vi "Programa Vent.vi"() -> ()   [LabVIEW 2021]
uses:
  TabControl.ctl
  4c7040a6-f012-4fa6-bc11-eaa48d4a9fce.vi
  <vilib>/Utility/file.llb/Write Delimited Spreadsheet (DBL).vi
  <vilib>/Instr/_visa.llb/VISA Configure Serial Port (Instr).vi
panel:
  out "Fecha y Hora":timestamp=timestamp(3714054510.5922894 s since 1904-01-01) format="%<%X\n%x>T"
  in  "Modo Operación":bool=TRUE
  in  "Comenzar Respiración":bool
  in  "Modo Asistido":bool
  in  "stop":bool
  in  "Tab Control 2":T1
  out "MV":i16=211
  out "PEEP":i16=4
  out "FLUJO":i16
  out "VOLUMEN":i16=211
  in  "Porcentaje \nde flujo (%)":i32=55 min=0 max=100 step=1
  in  "PEEP":i32 min=0 max=20 step=1
  in  "Presión de Soporte":i32=15 min=10 max=60 step=1
  in  "Volumen":i32=350 min=100 max=2000 step=10
  in  "Tiempo Plateau":i32=500 min=0 max=1 step=1
  in  "Tiempo Espiración":i32=3 min=1 max=10 step=1
  out "PRESIÓN":waveform(dbl)(graph)
  out "T. CICLO":dbl=9.2 format="%#_2g"
  out "BPM":i16=7
  out "PIP":i16=1
  out "FLUJO":waveform(dbl)(graph)
  in  "(PC) Tiempo de inspiración":i32=3 min=1 max=10 step=1
  out "FLUJO 2":waveform(dbl)(graph)
  out "PRESIÓN 2":waveform(dbl)(graph)
  out "DiffPres":waveform(dbl)(graph)
  in  "PWM":bool
  in  "PEEP":bool
  in  "PRESIÓN":bool
  in  "Data storage":bool
  out "Serial Read":string="Presion: 1.42,Peep: 3.57,Presion_soporte: 20,Flujo: -0.35,Volumen deseado: 350, Volumen inspiracion: 211.01,PIP: 1.00,VEF: 1.00,VIF: 211.00,T_muestreo: 4.00, PWM Out: 5000, Timer_Count_0: 0, Etapa_Res: 0, Derivada_Presion: 0.00, duracion_ciclo: 9200.00, BPM: 6.52, PWM_Caract: 0, T. Trans_Caract: 0.00, MV: 0.00, String: 0.000000,50.000000,20.000000,5.000000,350.000000,3000.000000,500.000000,0.000000,0.000000,0.000000,0.000000\r\r\n"
  out "Serial Write":string="0.000000,50.000000,20.000000,5.000000,350.000000,3000.000000,500.000000,0.000000,0.000000,0.000000,0.000000\r\n"
  in  "Caract. Escalon":bool
  in  "Caract. Rampa":bool
  in  "Comenzar Caracterizacion":bool
  in  "KI":i32=45 min=0 max=100 step=1
  in  "KP":i32=100 min=0 max=1000 step=1
  out "TIEMPO \nDE CICLO":dbl
  out "PRESIÓN SOPORTE\n (DEBUGGING)":dbl
  out "ETAPA \nRESPIRATORIA":dbl
  out "ERROR (PC)":dbl
  out "PWM \nCARACTERIZACIÓN":dbl
  out "PWM OUT":dbl
  in  "Caract. Pulmón":bool
  in  "Ruta de archivo":path=path "C:/Users/arakh/Desktop/MejoraVI/CalibTeensy.txt"
  in  "PRESIÓN MAX.":i32=30 min=0 max=100 step=1
  in  "PEEP MAX.":i32=30 min=0 max=100 step=1
  in  "RAPIDEZ APERTURA %":i32=30 min=0 max=100 step=1
  out "DeltaPDecay":waveform(dbl)(graph)
  out "PWM Out":waveform(dbl)(graph)
  # "Modo de Operación"
  # "INICIO"
  # "Funciones"
  # "GRÁFICOS"
  # "AJUSTES"
  # "AVANZADO"
  # "Ventilador Mecánico de Emergencia UTP-100P v5"
  # "PARÁMETROS FUNCIONALES"
  # "Porcentaje \nde flujo (%)"
  # "PEEP\n (cm H2O)"
  # "GRÁFICOS"
  # "PC: Tiempo de insp.  (seg.)"
  # "Presión de \nsoporte \n(cm H2O)"
  # "Volumen(ml)"
  # "Tiempo de esp. (seg.)"
  # "Tiempo de plateau (miliseg.)"
  # "tiempo"
  # "GRÁFICOS"
  # "PRESIÓN (cm H20)"
  # "Tiempo"
  # "AJUSTES"
  # "CARACTERIZACIÓN\n DE VÁLVULA"
  # "(PC) AJUSTES DE CONTROLADOR"
  # "ALMACENAMIENTO\nDE DATOS"
  # "CARACTERIZACIÓN \nDE PULMÓN"
  # "* Varía los parámetros incrementalmente por cada ciclo respiratorio."
  # "DATOS TEENSY"
  # "Seccion de Datos:"
  # "AJUSTES AVANZADOS"
  # "Delta P Decay (Diff)"
  # "PWM out"
  # "Tiempo"
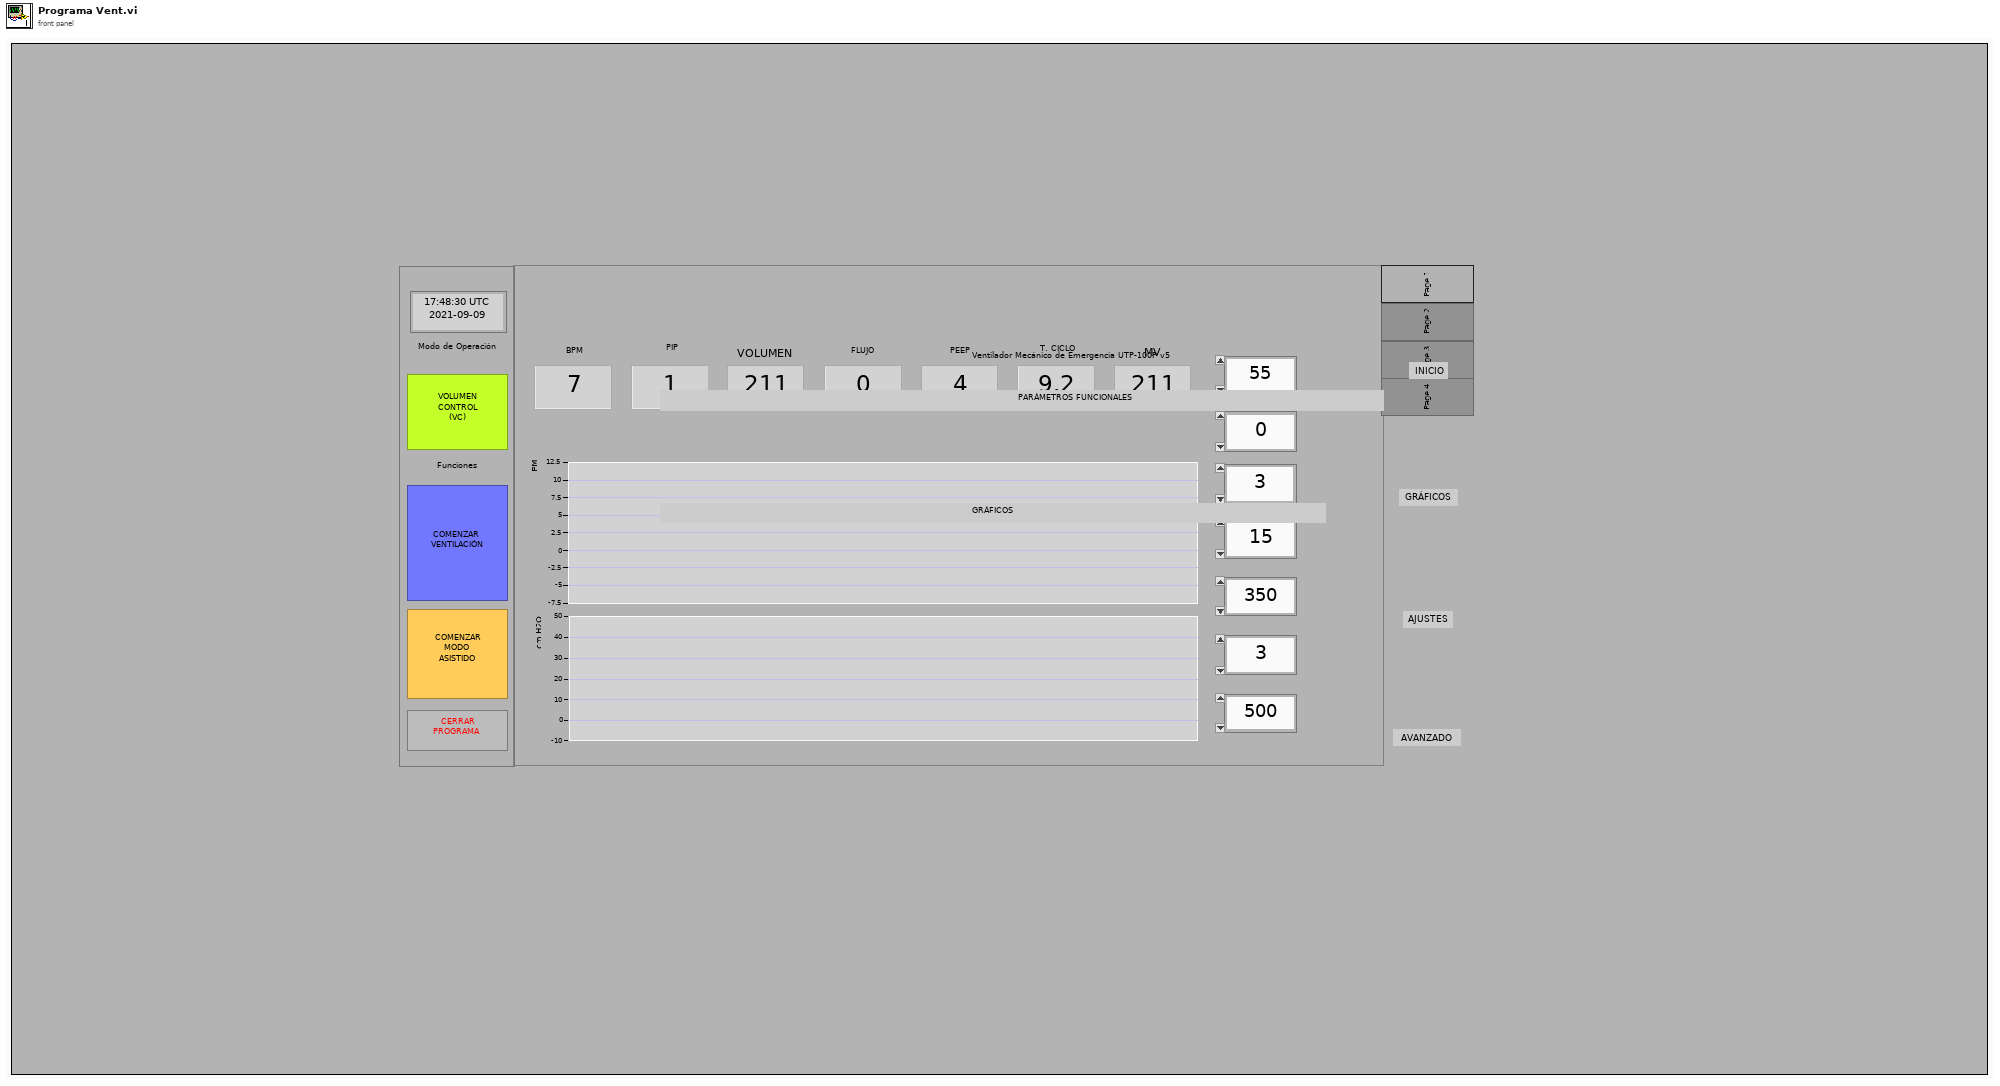
[diagram p1: front panel]
types:
  T1 = typedef "TabControl.ctl" = enum32{"Page 1", "Page 2", "Page 3", "Page 4"}
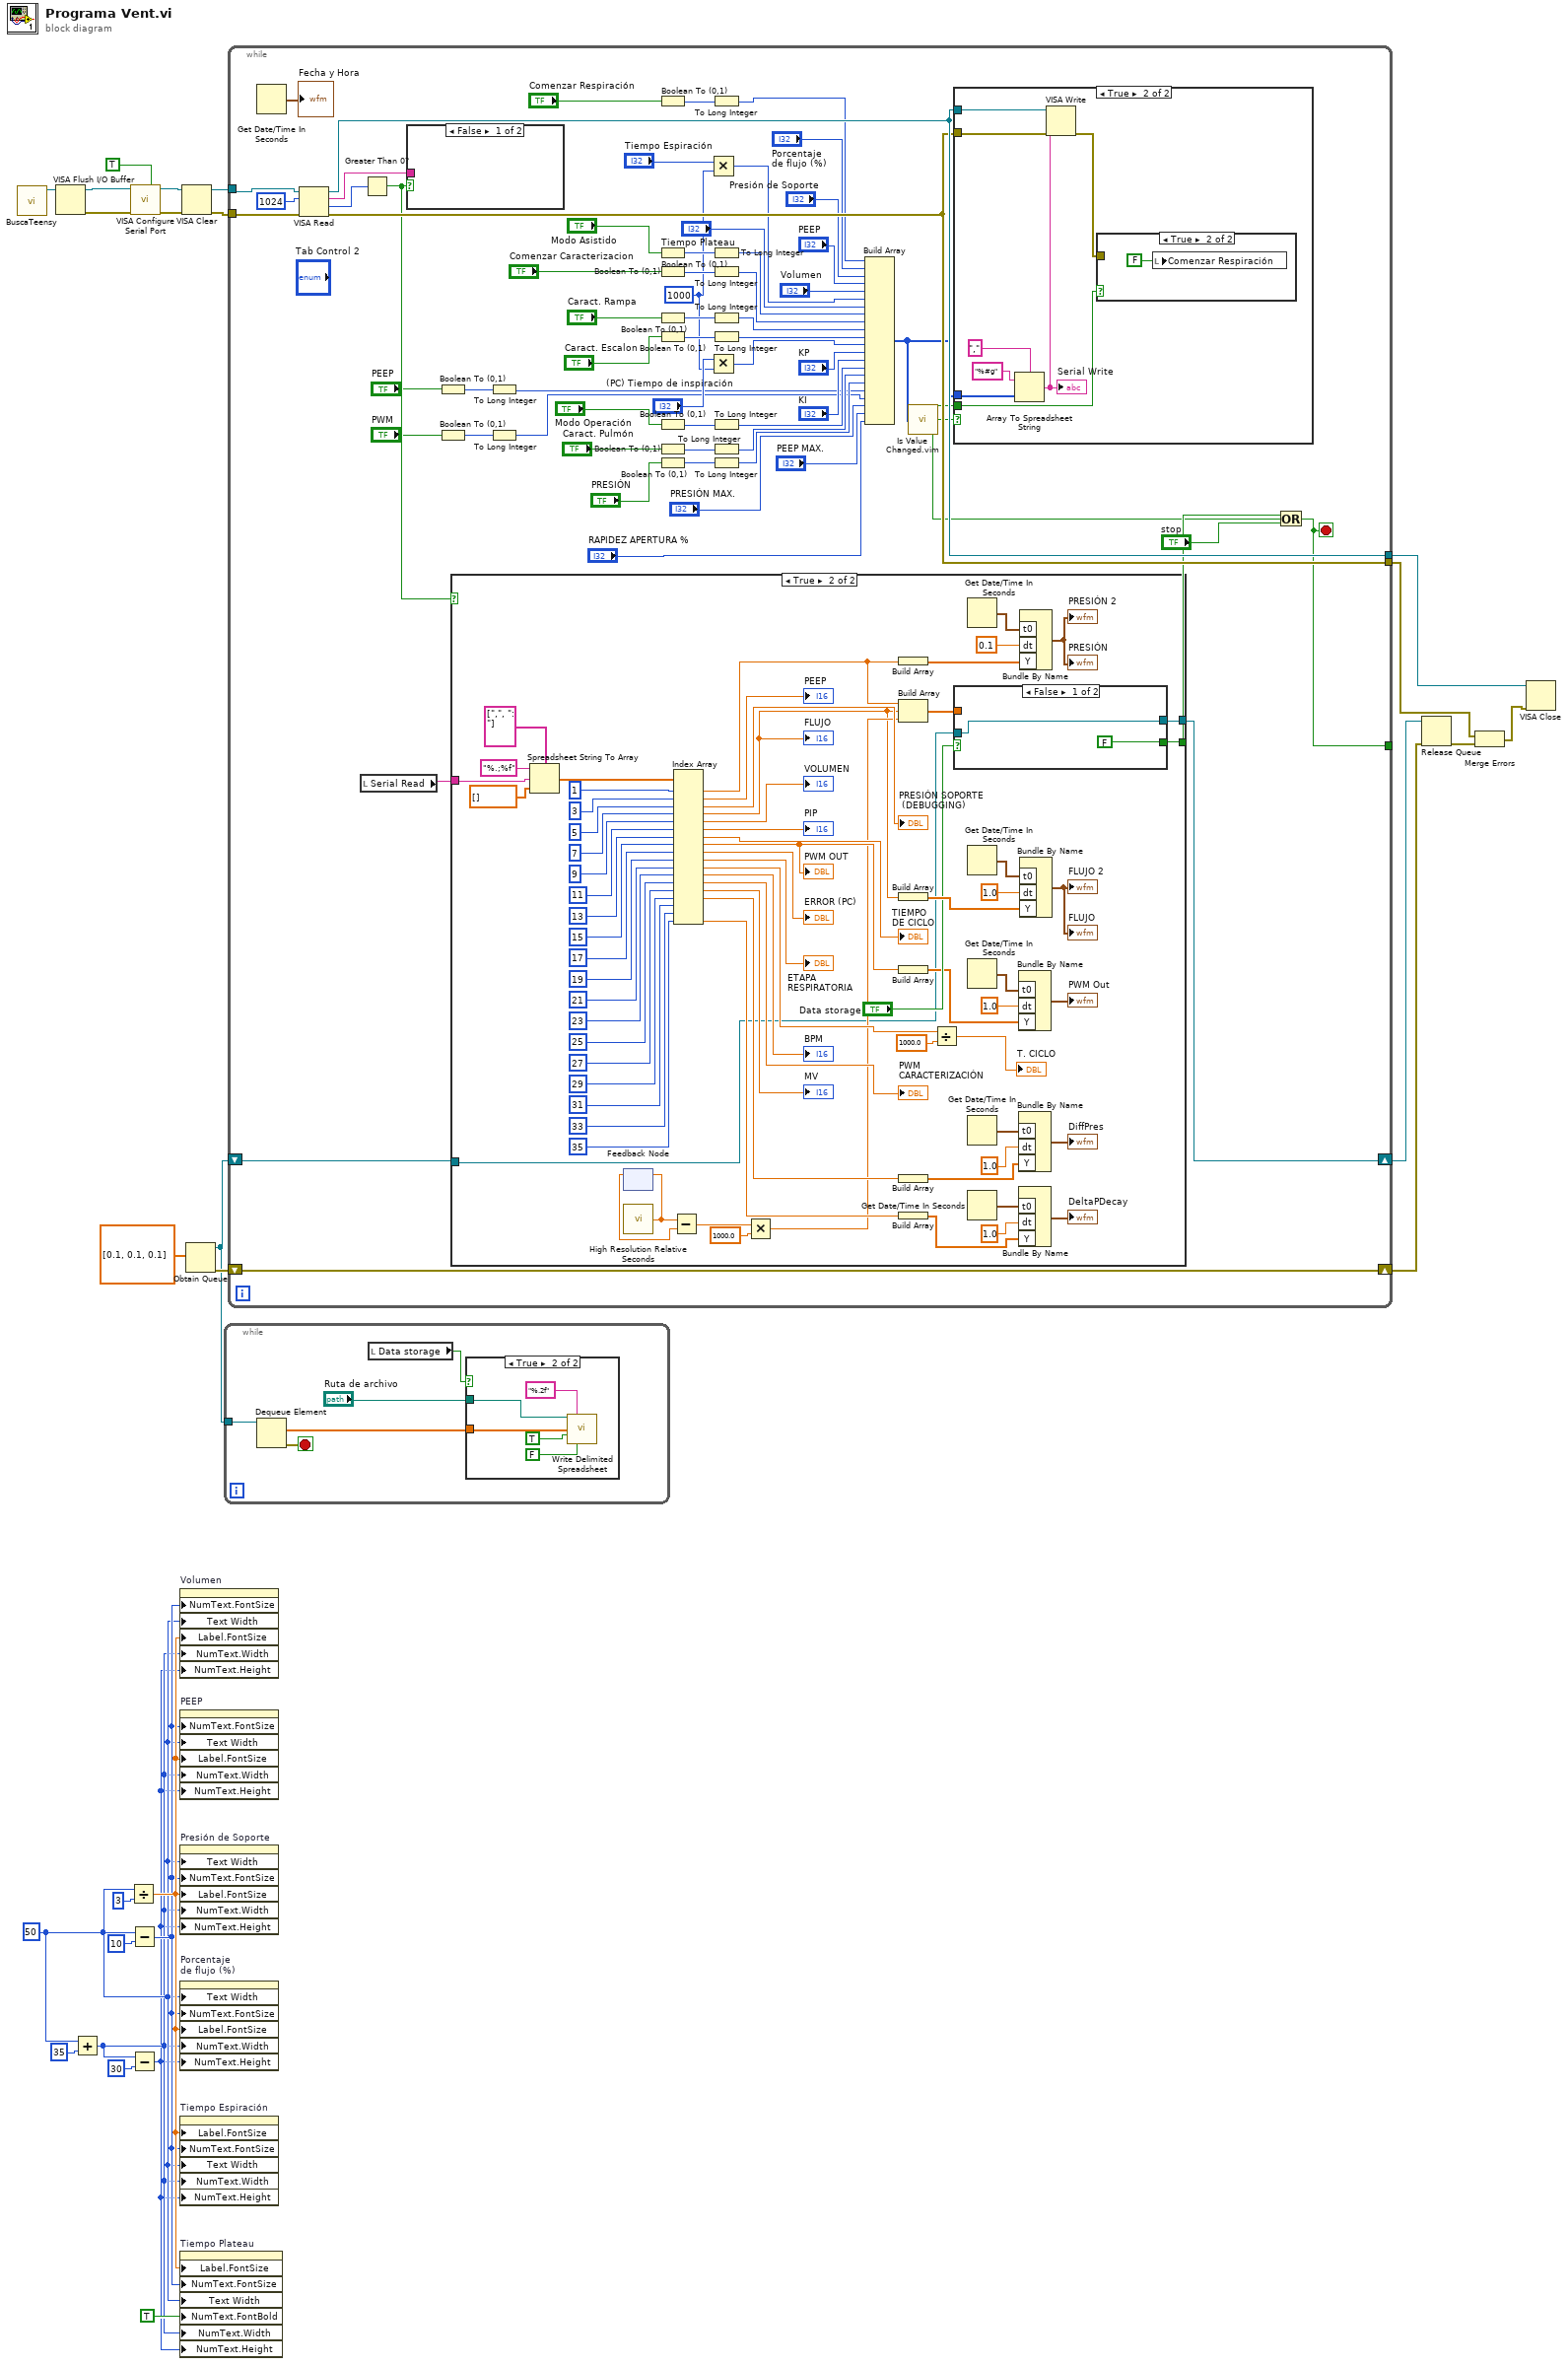
[diagram p0: block diagram]
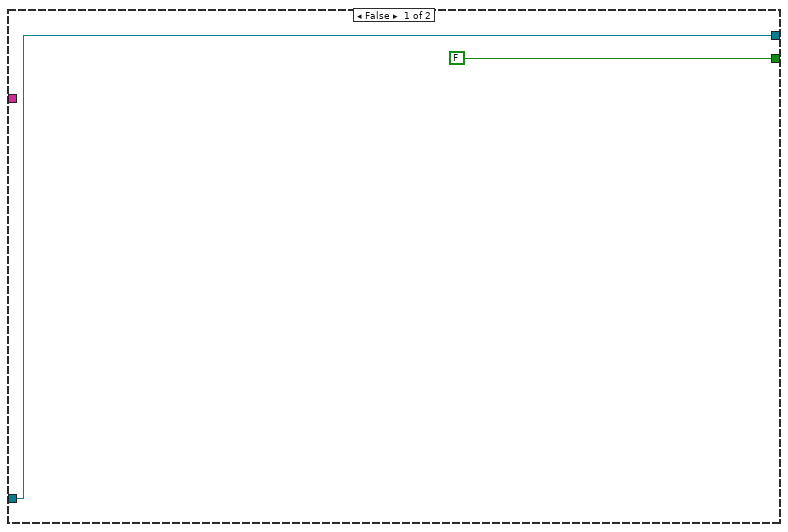
[diagram p3: hidden frame]
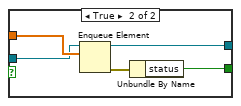
[diagram p4: hidden frame]
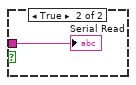
[diagram p5: hidden frame]
diagram:
  w14 = u32 50 ("Numeric Text.Size:Height")
  n1 = call "BuscaTeensy.vi"() -> ("VISA resource name out"=w19:refnum<visa-resource-name>)  [unwired: 15 in]
  n2 = VISA Flush I/O Buffer(VISA resource name=w19) -> (VISA resource name out=w21:refnum<visa-resource-name>, error out=w20:errorcluster)  [unwired: 2 in]
  n3 = Add(x=w14, y=u32 35) -> (x+y=w12:u32)
  n4 = Divide(x=w14, y=u32 3) -> (x/y=w16:dbl)
  n5 = Subtract(x=w14, y=u32 10 ("x")) -> (x-y=w15:u32)
  n6 = Subtract(x=w12, y=u32 30) -> (x-y=w10:u32)
  n7 = call-poly "VISA Configure Serial Port"("VISA resource name"=w21, "Enable Termination\nChar (T)"=TRUE ("Enable Termination\nChar (T)"), "error in (no error)"=w20) -> ("VISA resource name out"=w25:refnum<visa-resource-name>, "error out"=w24:errorcluster)  [unwired: 11 in]
  n8 = property on="Volumen" class="DigNum (strict)"("NumText.FontSize"=w15, "Text Width"=w14, "Label.FontSize"=w16, "NumText.Width"=w12, "NumText.Height"=w10) -> ()  [unwired: 2 in, 2 out]
  n9 = property on="PEEP" class="DigNum (strict)"("NumText.FontSize"=w15, "Text Width"=w14, "Label.FontSize"=w16, "NumText.Width"=w12, "NumText.Height"=w10) -> ()  [unwired: 2 in, 2 out]
  n10 = property on="Presión de Soporte" class="DigNum (strict)"("Text Width"=w14, "NumText.FontSize"=w15, "Label.FontSize"=w16, "NumText.Width"=w12, "NumText.Height"=w10) -> ()  [unwired: 2 in, 2 out]
  n11 = property on="Porcentaje \nde flujo (%)" class="DigNum (strict)"("Text Width"=w14, "NumText.FontSize"=w15, "Label.FontSize"=w16, "NumText.Width"=w12, "NumText.Height"=w10) -> ()  [unwired: 2 in, 2 out]
  n12 = property on="Tiempo Espiración" class="DigNum (strict)"("Label.FontSize"=w16, "NumText.FontSize"=w15, "Text Width"=w14, "NumText.Width"=w12, "NumText.Height"=w10) -> ()  [unwired: 2 in, 2 out]
  n13 = property on="Tiempo Plateau" class="DigNum (strict)"("Label.FontSize"=w16, "NumText.FontSize"=w15, "Text Width"=w14, "NumText.FontBold"=TRUE ("Numeric Text.Font:Bold"), "NumText.Width"=w12, "NumText.Height"=w10) -> ()  [unwired: 2 in, 2 out]
  n14 = VISA Clear(VISA resource name=w25, error in (no error)=w24) -> (VISA resource name out=w23:refnum<visa-resource-name>, error out=w22:errorcluster)
  n15 = Obtain Queue(element data type=dbl[] [0.1, 0.1, 0.1]) -> (queue out=w4:refnum<queue>, error out=w6:errorcluster)  [unwired: 4 in, 1 out]
  n16 = while {
    tunnel: w4 -> [w29]
    stop <- w30 stop-if-true
    n17 = Dequeue Element(queue=w29) -> (element=w31:dbl[], error out=w30:errorcluster)  [unwired: 2 in, 2 out]
    n18 = local read "Data storage"() -> (w32:bool)
    n19 = case shown="True" w32 {
      tunnel: w31 -> [_ w34]
      tunnel: "Ruta de archivo" -> [_ w33]
      frame False {
      }
      frame True {
        n20 = call-poly <vilib>:"Write Delimited Spreadsheet.vi"("file path (dialog if empty)"=w33, "format (%.3f)"="%.2f", "1D data"=w34, "append to file? (new file:F)"=TRUE, "transpose? (no:F)"=FALSE) -> ()  [unwired: 9 in, 2 out]
      }
    }
  }
  n21 = while {
    tunnel: [w98] -> w26
    tunnel: [w97] -> w2
    tunnel: w23 -> [w96]
    tunnel: w22 -> [w95]
    tunnel: [w40] -> _
    shift-right: [w39] -> w5
    shift-left: w6 -> [w39]
    shift-right: [w43] -> w7
    shift-left: w4 -> [w44]
    stop <- w40 stop-if-true
    w69 = 1000 ("y")
    n22 = Get Date/Time In Seconds() -> (seconds since 1Jan1904=→"Fecha y Hora":timestamp)
    n23 = VISA Read(VISA resource name=w96, byte count=u32 1024, error in (no error)=w95) -> (VISA resource name out=w98:refnum<visa-resource-name>, read buffer=w100:string, return count=w93:u32, error out=w97:errorcluster)
    n24 = local read "Serial Read"() -> (w99:string)
    n25 = Greater Than 0?(x=w93) -> (x > 0?=w92:bool)
    n26 = case shown="False" w92 {
      tunnel: w100 -> [_ w181]
      frame False {
      }
      frame True {
        "Serial Read" <- w181
      }
    }
    n27 = Boolean To (0,1)(Boolean="PEEP") -> (0, 1=w53:i16)
    n28 = Boolean To (0,1)(Boolean="PWM") -> (0, 1=w52:i16)
    n29 = case shown="True" w92 {
      tunnel: w99 -> [_ w170]
      tunnel: w44 -> [w101 w106]
      tunnel: [w101 w105] -> w43
      tunnel: [FALSE ("status") w104] -> w41
      frame False {
      }
      frame True {
        n30 = Spreadsheet String To Array(delimiter (Tab)=string[] [",", ": "], format string="%.;%f", spreadsheet string=w170, array type (2D Dbl)=dbl[] []) -> (array=w169:dbl[])
        n31 = feedback #1() -> (w124:dbl)  [unwired: 1 in]
        n32 = call <vilib>:"High Resolution Relative Seconds.vi"() -> ("relative seconds"=w125:dbl)
        n33 = feedback-in #1(w125) -> ()
        n34 = Subtract(x=w125, y=w124) -> (x-y=w123:dbl)
        n35 = Index Array(array=w169, index #1=1 ("index"), index #2=3 ("index"), index #3=5 ("index"), index #4=7 ("index"), index #5=9 ("index"), index #6=11 ("index"), index #7=13 ("index"), index #8=15 ("index"), index #9=17 ("index"), index #10=19 ("index"), index #11=21 ("index"), index #12=23 ("index"), index #13=25 ("index"), index #14=27 ("index"), index #15=29 ("index"), index #16=31 ("index"), index #17=33 ("index"), index #18=35 ("index")) -> (element #1=w128:dbl, element #2=→"PEEP":dbl, element #3=→"PRESIÓN SOPORTE\n (DEBUGGING)":dbl, element #4=w103:dbl, element #5=→"VOLUMEN":dbl, element #6=→"PIP":dbl, element #7=→"TIEMPO \nDE CICLO":dbl, element #8=w130:dbl, element #9=→"ERROR (PC)":dbl, element #10=→"ETAPA \nRESPIRATORIA":dbl, element #11=w138:dbl, element #12=→"BPM":dbl, element #13=→"PWM \nCARACTERIZACIÓN":dbl, element #14=→"MV":dbl, element #15=w129:dbl, element #18=w126:dbl)  [unwired: 2 out]
        "FLUJO" <- w103
        "PWM OUT" <- w130
        n36 = Multiply(x=w123, y=1000.0) -> (x*y=w121:dbl)
        n37 = Build Array(w128) -> (w147:dbl[])
        n38 = Build Array(w128, w103, w121) -> (w133:dbl[])
        n39 = Build Array(w103) -> (w146:dbl[])
        n40 = Build Array(w130) -> (w131:dbl[])
        n41 = Build Array(w129) -> (w112:dbl[])
        n42 = Build Array(w126) -> (w109:dbl[])
        n43 = Divide(x=w138, y=1000.0) -> (x/y=→"T. CICLO":dbl)
        n44 = case shown="False" "Data storage" {
          tunnel: w133 -> [_ w180]
          tunnel: w106 -> [w174 w179]
          tunnel: [w174 w178] -> w105
          tunnel: [FALSE ("status") w176] -> w104
          frame False {
          }
          frame True {
            n45 = Enqueue Element(queue=w179, element=w180) -> (queue out=w178:refnum<queue>, error out=w177:errorcluster)  [unwired: 2 in, 1 out]
            n46 = Unbundle By Name(w177) -> ("status"=w176:bool)
          }
        }
        n47 = Get Date/Time In Seconds() -> (seconds since 1Jan1904=w149:timestamp)
        n48 = Get Date/Time In Seconds() -> (seconds since 1Jan1904=w120:timestamp)
        n49 = Get Date/Time In Seconds() -> (seconds since 1Jan1904=w117:timestamp)
        n50 = Get Date/Time In Seconds() -> (seconds since 1Jan1904=w114:timestamp)
        n51 = Get Date/Time In Seconds() -> (seconds since 1Jan1904=w107:timestamp)
        n52 = Bundle By Name("t0"=w117, "dt"=1.0, "Y"=w131) -> (→"PWM Out":waveform(dbl))  [unwired: 1 in]
        n53 = Bundle By Name("t0"=w114, "dt"=1.0, "Y"=w112) -> (→"DiffPres":waveform(dbl))  [unwired: 1 in]
        n54 = Bundle By Name("t0"=w107, "dt"=1.0, "Y"=w109) -> (→"DeltaPDecay":waveform(dbl))  [unwired: 1 in]
        n55 = Bundle By Name("t0"=w149, "dt"=0.1, "Y"=w147) -> (→"PRESIÓN" →"PRESIÓN 2":waveform(dbl))  [unwired: 1 in]
        n56 = Bundle By Name("t0"=w120, "dt"=1.0, "Y"=w146) -> (→"FLUJO" →"FLUJO 2":waveform(dbl))  [unwired: 1 in]
      }
    }
    n57 = To Long Integer(number=w53) -> (32bit integer=w48:i32)
    n58 = To Long Integer(number=w52) -> (32bit integer=w47:i32)
    n59 = Boolean To (0,1)(Boolean="Comenzar Respiración") -> (0, 1=w81:i16)
    n60 = Boolean To (0,1)(Boolean="Modo Asistido") -> (0, 1=w79:i16)
    n61 = Boolean To (0,1)(Boolean="Comenzar Caracterizacion") -> (0, 1=w78:i16)
    n62 = Boolean To (0,1)(Boolean="Caract. Rampa") -> (0, 1=w77:i16)
    n63 = Boolean To (0,1)(Boolean="Caract. Escalon") -> (0, 1=w76:i16)
    n64 = Boolean To (0,1)(Boolean="Modo Operación") -> (0, 1=w62:i16)
    n65 = Boolean To (0,1)(Boolean="Caract. Pulmón") -> (0, 1=w57:i16)
    n66 = Boolean To (0,1)(Boolean="PRESIÓN") -> (0, 1=w54:i16)
    n67 = Multiply(x="Tiempo Espiración", y=w69) -> (x*y=w70:i32)
    n68 = Multiply(x="(PC) Tiempo de inspiración", y=w69) -> (x*y=w74:i32)
    n69 = To Long Integer(number=w81) -> (32bit integer=w80:i32)
    n70 = To Long Integer(number=w79) -> (32bit integer=w68:i32)
    n71 = To Long Integer(number=w78) -> (32bit integer=w67:i32)
    n72 = To Long Integer(number=w77) -> (32bit integer=w66:i32)
    n73 = To Long Integer(number=w76) -> (32bit integer=w65:i32)
    n74 = To Long Integer(number=w62) -> (32bit integer=w60:i32)
    n75 = To Long Integer(number=w57) -> (32bit integer=w56:i32)
    n76 = To Long Integer(number=w54) -> (32bit integer=w49:i32)
    n77 = Build Array(w80, "Porcentaje \nde flujo (%)", "Presión de Soporte", "PEEP", "Volumen", w70, "Tiempo Plateau", w68, w67, w66, w65, w74, "KP", "KI", w60, w56, w49, w48, w47, "PRESIÓN MAX.", "PEEP MAX.", "RAPIDEZ APERTURA %") -> (w83:i32[])
    n78 = call "Is Value Changed.vim"("value"=w83) -> ("changed or first call?"=w91:bool)
    n79 = Or(x=w41, y="stop") -> (x .or. y?=w40:bool)
    n80 = case shown="True" w91 {
      tunnel: w98 -> [_ w187]
      tunnel: w97 -> [_ w186]
      tunnel: w83 -> [_ w185]
      tunnel: w40 -> [_ w183]
      frame False {
      }
      frame True {
        n81 = Array To Spreadsheet String(delimiter (Tab)=",", array=w185, 3:"%#g" ("format string")) -> (spreadsheet string=w182:string)
        "Serial Write" <- w182
        n82 = VISA Write(VISA resource name=w187, write buffer=w182, error in (no error)=w186) -> (error out=w184:errorcluster)  [unwired: 2 out]
        n83 = case shown="True" w183 {
          tunnel: w184 -> [_ _]
          frame False {
          }
          frame True {
            n84 = local write "Comenzar Respiración"(FALSE ("Comenzar Respiración")) -> ()
          }
        }
      }
    }
  }
  n85 = Release Queue(queue=w7, error in (no error)=w5) -> (error out=w3:errorcluster)  [unwired: 1 in, 2 out]
  n86 = Merge Errors(w2, w3) -> (w1:errorcluster)
  n87 = VISA Close(VISA resource name=w26, error in (no error)=w1) -> ()  [unwired: 1 out]
